vi "ProcessBufferUpdatesSubnet2.vi"(11 "MockFAILC2Settings":T1={"ModbusTxDataFIFO"="MockbusPort2TxFIFO", "Code17Memory"="MockFAILC2Code17", "BufferUpdateFIFO"="MockFAILC2Command", "ModbusRxDataFIFO"="MockbusPort2RxFIFO", "Code18Memory"="MockFAILC2Code18", "Code65Memory"="MockFAILC2Code65", "Code66Memory"="MockFAILC2Code66", "Code67Memory"="MockFAILC2Code67", "Code72Memory"="MockFAILC2Code72", "Code80Memory"="MockFAILC2Code80", "Code110Memory"="MockFAILC2Code110", "CRCDataFIFO"="MockFAILC2CRCDataFIFO", "CRCCalculateFIFO"="MockFAILC2CRCCalculateFIFO", "CRCFIFO"="MockFAILC2CRCFIFO"}) -> ()   [LabVIEW 2016]
uses:
  DataTypes/MockFAILC2Settings.ctl
  FPGAMockHPILC/DataTypes/MockHPBufferUpdateLoopData.ctl
  FPGAMockHPILC/DataTypes/MockHPBufferUpdateStates.ctl
  <vilib>/Platform/TimedLoop/XDataNode/timing_clust.ctl
  <vilib>/Platform/TimedLoop/XDataNode/nitl_modes.ctl
  <vilib>/Platform/TimedLoop/XDataNode/wakeup.ctl
  <vilib>/rvi/Emulation/niFpgaSctlEmulationGetInTimedLoop.vi
  <vilib>/rvi/Emulation/niFpgaEmulationReportErrorSimple.vi
  <vilib>/rvi/Emulation/niFpgaGetClockAttributes.vi
  <vilib>/rvi/Emulation/niFpgaCriticalErrorInLSC.vi
  <vilib>/rvi/DataTransferAndStorage/Container/Common/niFpgaContainerExecOnDevCompGetState.vi
  <vilib>/rvi/Emulation/niFpgaEmulationIsFPGAContextNoSignature.vi
  <vilib>/rvi/errors/niFpgaSetErrorForExecOnDevCompSimple.vi
  <vilib>/rvi/eio/common/nirviEmuReportErrorAndStop.vi
  <vilib>/rvi/DataTransferAndStorage/Container/Common/niFpgaContainerGetUniqueNameForEmu.vi
  <vilib>/rvi/FIFO/Fifo_Resource/nirvififoEmulationSetSize.vi
  <vilib>/rvi/FIFO/Fifo_Resource/nirviFifoEmulationQueueMgr.vi
  <instcachedir>/0/nirviFifoEmulationQueueMgr_E5CAEC123FF24DC58D834DCA3CDAA9B5.lvgen/nirviFifoEmulationQueueMgr_E5CAEC123FF24DC58D834DCA3CDAA9B5_009.vi
  <vilib>/rvi/FIFO/Fifo_Resource/nirvififoEmulationDetermineInputValidOut.vi
  <vilib>/rvi/FIFO/Fifo_Resource/nirvififoEmulationCreateLock.vi
  <vilib>/rvi/Emulation/niFpgaProcessEmulError.vi
  <vilib>/rvi/FIFO/Fifo_Resource/nirvififoEmulationObtainLock.vi
  <vilib>/rvi/FIFO/Fifo_Resource/nirvififoEmulationReleaseLock.vi
  <vilib>/rvi/occurrence/nirviWaitOnOccurrenceBase.vi
  <vilib>/rvi/errors/nirviReportUnexpectedCaseInternalError.vi
  <vilib>/rvi/errors/nirviReportUnexpectedCaseInternalError (U32).vi
  <vilib>/Utility/error.llb/Clear Errors.vi
  <vilib>/rvi/interface/RandomDataEmulation/niFpgaRandomDataHandleErrors.vi
  <vilib>/rvi/Memory/Memory_Emulation/niFpgaMemoryEmulationCacheClearOnFirstRun.vi
  <vilib>/rvi/Memory/Memory_Emulation/nirvimemoryEmulationManagerCache_MakeExclusive.vi
  <vilib>/rvi/Memory/Memory_Emulation/niFpgaMemoryEmulationValidateCache.vi
  <vilib>/rvi/Memory/Memory_Emulation/nirvimemoryEmulationManagerCache_InsertValue.vi
  <vilib>/rvi/Memory/Memory_Emulation/nirvimemoryEmulationManagerCache_ReleaseExclusive.vi
  <vilib>/rvi/Memory/Memory_Emulation/nirvimemoryEmulationManagerCache_GetValue.vi
  <vilib>/rvi/Memory/Memory_Emulation/nirvimemoryEmulationManagerCache_SetValue.vi
  <vilib>/rvi/Emulation/niFpgaSctlEmulationResourceMgr.vi
  <vilib>/Platform/TimedLoop/XDataNode/XDataNode.xnode
  <vilib>/rvi/DataTransferAndStorage/Container/XNode/niFpgaContainer.xnode
  <vilib>/rvi/FIFO/Fifo_Resource/niFpgaFifoEmulationRefIn.vi
  <vilib>/rvi/Memory/Memory_Emulation/niFpgaMemoryEmulationRefIn.vi
  <vilib>/Platform/TimedLoop/XDataNode/XDNodeRunTimeDep.lvlib
  FPGAMockHPILC/FPGAMockHPILC.lvlib
  FPGAMockFAILC.lvlib
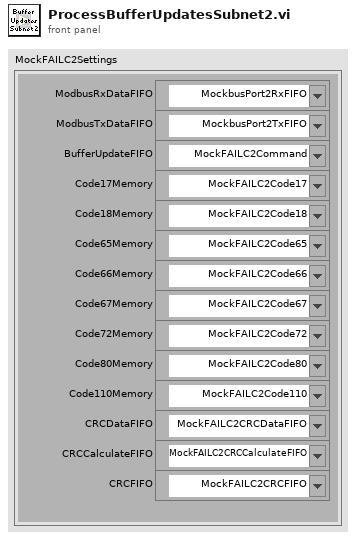
[diagram p1: front panel]
types:
  T1 = typedef "FPGAMockFAILC.lvlib/MockFAILC2Settings.ctl" = cluster{"ModbusTxDataFIFO":refnum<k21>, "Code17Memory":refnum<k21>, "BufferUpdateFIFO":refnum<k21>, "ModbusRxDataFIFO":refnum<k21>, "Code18Memory":refnum<k21>, "Code65Memory":refnum<k21>, "Code66Memory":refnum<k21>, "Code67Memory":refnum<k21>, "Code72Memory":refnum<k21>, "Code80Memory":refnum<k21>, "Code110Memory":refnum<k21>, "CRCDataFIFO":refnum<k21>, "CRCCalculateFIFO":refnum<k21>, "CRCFIFO":refnum<k21>}
  T2 = typedef "FPGAMockHPILC.lvlib/MockHPBufferUpdateLoopData.ctl" = cluster{"BufferUpdateLoopStates":T3, "Address":u8, "Function":u8, "Length":u8, "Data":u8, "Index":u8}
  T3 = typedef "FPGAMockHPILC.lvlib/MockHPBufferUpdateStates.ctl" = enum16{"ReadAddress", "ReadFunction", "ReadLength", "ReadData", "WriteData"}
  T4 = typedef "XDNodeRunTimeDep.lvlib/timing_clust.ctl" = cluster{"Expected End [f-1]":u64, "Actual End [f-1]":u64, "Finished Late? [f-1]":bool, "Expected End [i-1]":u64, "Actual End [i-1]":u64, "Finished Late? [i-1]":bool, "Expected Start [i]":u64, "Actual Start [i]":u64, "Expected Start [f]":u64, "Actual Start [f]":u64, "Source Name":string, "Structure Name":string, "Period":i64, "Deadline":i64, "Offset":i64, "Start":i64, "Priority":i32, "Timeout":i32, "Mode":T5, "Wakeup Reason":T6, "Error":errorcluster, "Source Type":string, "Secondary Source Type":string, "Global End Time":u64, "Global Start Time":u64, "Frame Duration":u64, "Iteration Duration":u64, "Assigned CPU":i32, "I/O Scan Engine Mode":u32}
  T5 = typedef "XDNodeRunTimeDep.lvlib/nitl_modes.ctl" = enum32{"No Change", "Process missed periods, maintain original phase", "Discard missed periods, maintain original phase", "Process missed periods, ignore original phase", "Discard missed periods, ignore original phase"}
  T6 = typedef "XDNodeRunTimeDep.lvlib/wakeup.ctl" = enum32{"Normal", "Aborted", "Asynchronous wakeup", "Timing source error", "Timed loop error", "Timeout"}
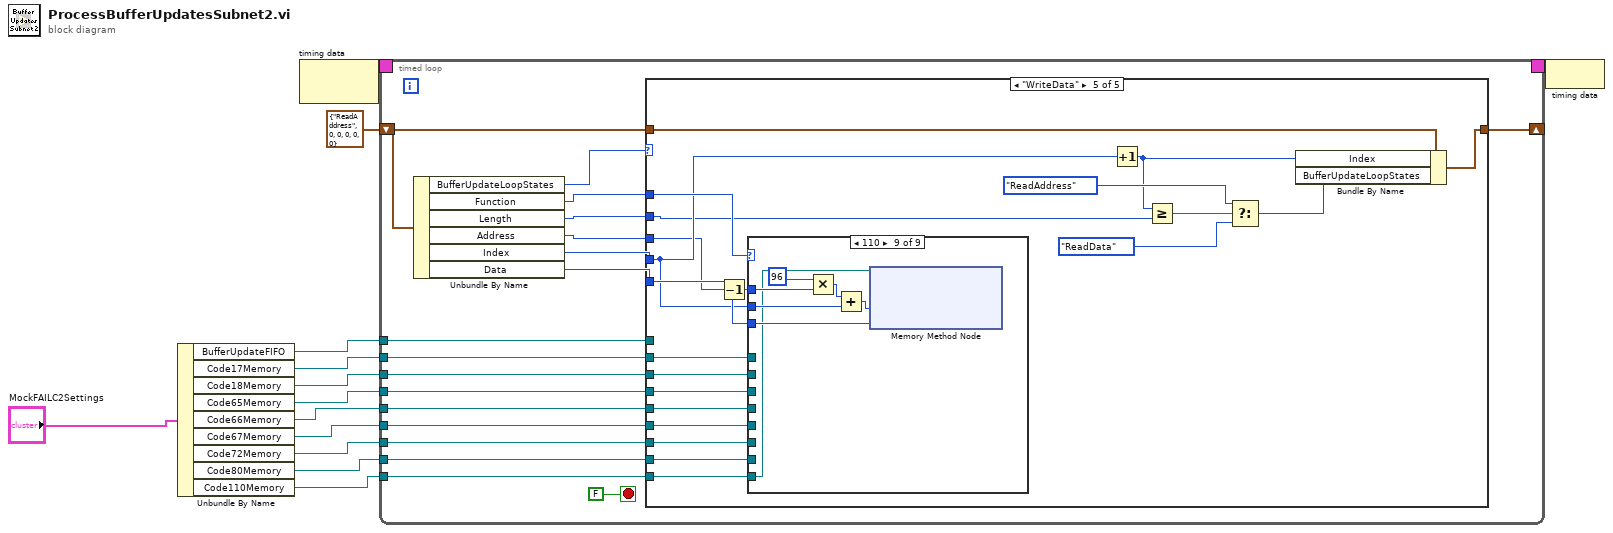
[diagram p0: block diagram]
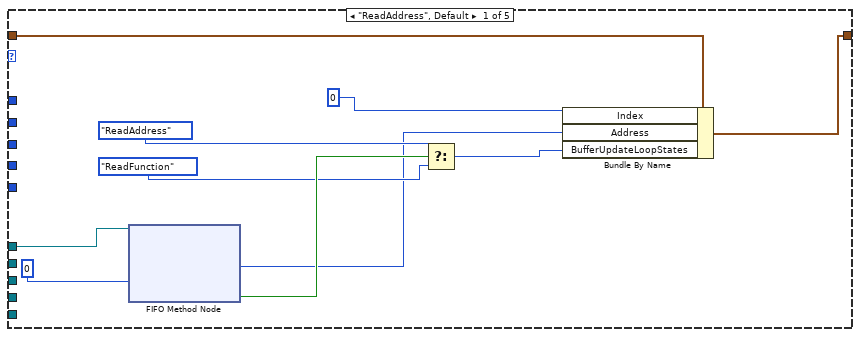
[diagram p2: hidden frame]
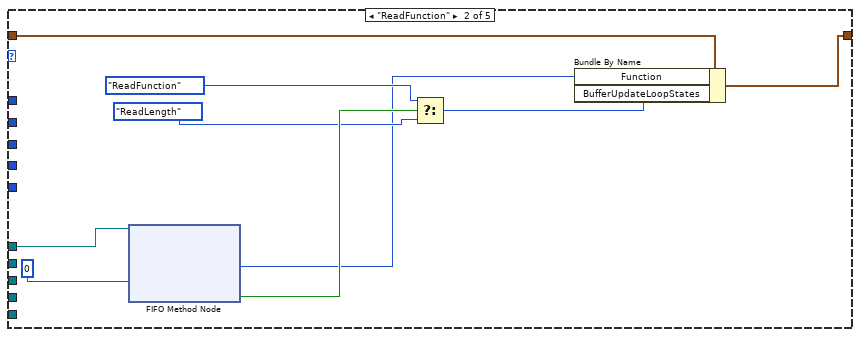
[diagram p3: hidden frame]
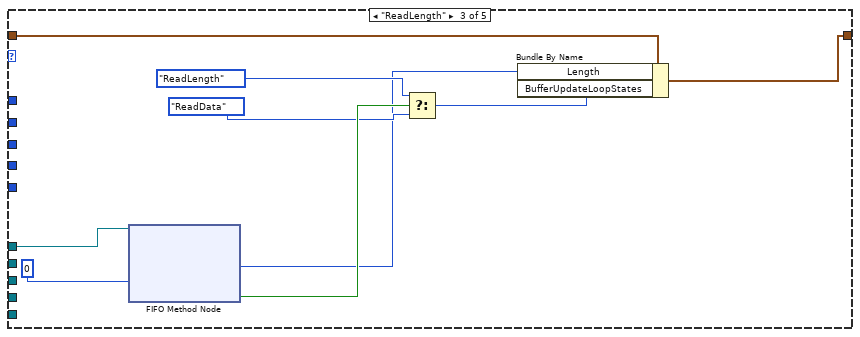
[diagram p4: hidden frame]
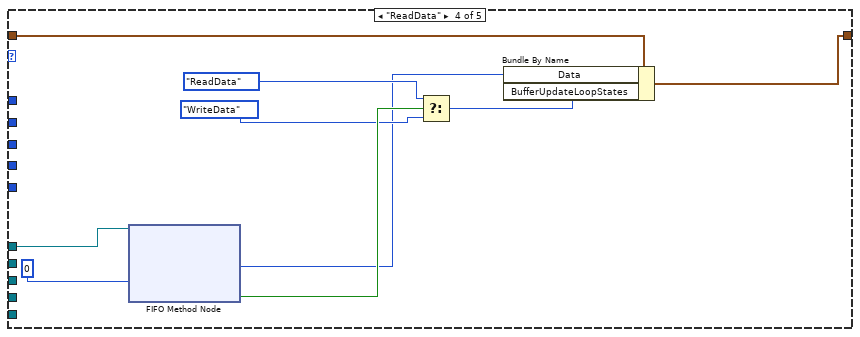
[diagram p5: hidden frame]
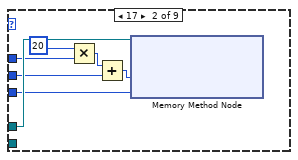
[diagram p7: hidden frame]
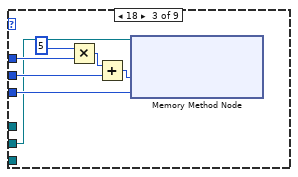
[diagram p8: hidden frame]
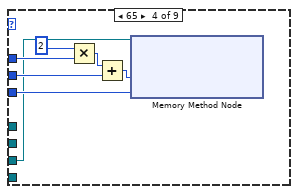
[diagram p9: hidden frame]
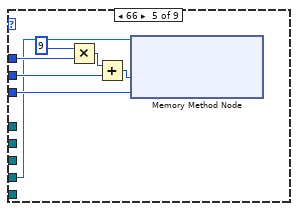
[diagram p10: hidden frame]
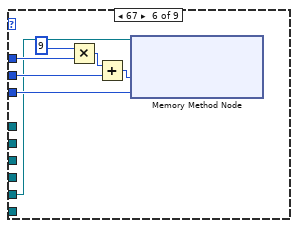
[diagram p11: hidden frame]
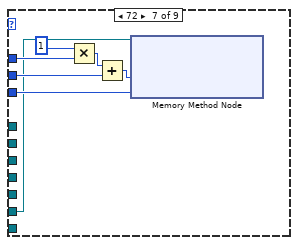
[diagram p12: hidden frame]
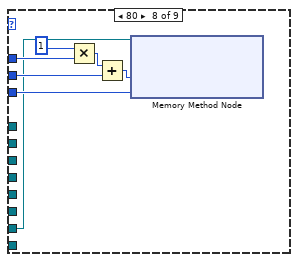
[diagram p13: hidden frame]
diagram:
  n1 = Unbundle By Name("MockFAILC2Settings") -> ("BufferUpdateFIFO"=w10:refnum<k21>, "Code17Memory"=w9:refnum<k21>, "Code18Memory"=w8:refnum<k21>, "Code65Memory"=w7:refnum<k21>, "Code66Memory"=w6:refnum<k21>, "Code67Memory"=w5:refnum<k21>, "Code72Memory"=w4:refnum<k21>, "Code80Memory"=w3:refnum<k21>, "Code110Memory"=w2:refnum<k21>)
  n2 = node-c288() -> (w13:T4)  [unwired: 1 in]
  n3 = timed-loop {
    timing: w13 -> [_]
    timing-out: [_] -> w12
    tunnel: w10 -> [w30]
    tunnel: w9 -> [w22]
    tunnel: w8 -> [w21]
    tunnel: w7 -> [w20]
    tunnel: w6 -> [w19]
    tunnel: w5 -> [w18]
    tunnel: w4 -> [w17]
    tunnel: w3 -> [w16]
    tunnel: w2 -> [w15]
    shift-right: [w24] -> _
    shift-left: T2 {"BufferUpdateLoopStates"=enum."ReadAddress", "Address"=0, "Function"=0, "Length"=0, "Data"=0, "Index"=0} ("MockHPBufferUpdateLoopData") -> [w29]
    stop <- FALSE stop-if-true
    n4 = Unbundle By Name(w29) -> ("BufferUpdateLoopStates"=w31:T3, "Function"=w28:u8, "Length"=w27:u8, "Address"=w26:u8, "Index"=w25:u8, "Data"=w23:u8)
    n5 = case shown="\"WriteData\"" w31 {
      tunnel: w30 -> [w41 w50 w59 w68 _]
      tunnel: w29 -> [w34 w43 w52 w61 w87]
      tunnel: w28 -> [_ _ _ _ w85]
      tunnel: w27 -> [_ _ _ _ w81]
      tunnel: w26 -> [_ _ _ _ w70]
      tunnel: w25 -> [_ _ _ _ w82]
      tunnel: [w33 w42 w51 w60 w86] -> w24
      tunnel: w23 -> [_ _ _ _ w83]
      tunnel: w22 -> [_ _ _ _ w84]
      tunnel: w21 -> [_ _ _ _ w77]
      tunnel: w20 -> [_ _ _ _ w76]
      tunnel: w19 -> [_ _ _ _ w75]
      tunnel: w18 -> [_ _ _ _ w74]
      tunnel: w17 -> [_ _ _ _ w73]
      tunnel: w16 -> [_ _ _ _ w72]
      tunnel: w15 -> [_ _ _ _ w71]
      frame "ReadAddress", Default {
        n6 = xnode ("FIFO Method Node")("Timeout"=0, "FIFO In"=w41) -> ("Element"=w36:u8, "Timed Out?"=w40:bool)  [unwired: 1 out]
        n7 = Select(t=MockHPBufferUpdateStates."ReadAddress" ("f"), s=w40, f=MockHPBufferUpdateStates."ReadFunction") -> (s? t:f=w35:T3)
        n8 = Bundle By Name(cluster=w34, "Index"=u8 0, "Address"=w36, "BufferUpdateLoopStates"=w35) -> (w33:T2)
      }
      frame "ReadFunction" {
        n9 = xnode ("FIFO Method Node")("Timeout"=0, "FIFO In"=w50) -> ("Element"=w45:u8, "Timed Out?"=w49:bool)  [unwired: 1 out]
        n10 = Select(t=MockHPBufferUpdateStates."ReadFunction" ("f"), s=w49, f=MockHPBufferUpdateStates."ReadLength") -> (s? t:f=w44:T3)
        n11 = Bundle By Name(cluster=w43, "Function"=w45, "BufferUpdateLoopStates"=w44) -> (w42:T2)
      }
      frame "ReadLength" {
        n12 = xnode ("FIFO Method Node")("Timeout"=0, "FIFO In"=w59) -> ("Element"=w54:u8, "Timed Out?"=w58:bool)  [unwired: 1 out]
        n13 = Select(t=MockHPBufferUpdateStates."ReadLength" ("f"), s=w58, f=MockHPBufferUpdateStates."ReadData") -> (s? t:f=w53:T3)
        n14 = Bundle By Name(cluster=w52, "Length"=w54, "BufferUpdateLoopStates"=w53) -> (w51:T2)
      }
      frame "ReadData" {
        n15 = xnode ("FIFO Method Node")("Timeout"=0, "FIFO In"=w68) -> ("Element"=w63:u8, "Timed Out?"=w67:bool)  [unwired: 1 out]
        n16 = Select(t=MockHPBufferUpdateStates."ReadData" ("f"), s=w67, f=MockHPBufferUpdateStates."WriteData") -> (s? t:f=w62:T3)
        n17 = Bundle By Name(cluster=w61, "Data"=w63, "BufferUpdateLoopStates"=w62) -> (w60:T2)
      }
      frame "WriteData" {
        n18 = Decrement(x=w70) -> (x-1=w69:u8)
        n19 = case shown="110" w85 {
          tunnel: w84 -> [_ w96 _ _ _ _ _ _ _]
          tunnel: w83 -> [_ w95 w103 w110 w117 w124 w131 w138 w145]
          tunnel: w82 -> [_ w93 w101 w108 w115 w122 w129 w136 w143]
          tunnel: w69 -> [_ w91 w99 w106 w113 w120 w127 w134 w141]
          tunnel: w77 -> [_ _ w97 _ _ _ _ _ _]
          tunnel: w76 -> [_ _ _ w104 _ _ _ _ _]
          tunnel: w75 -> [_ _ _ _ w111 _ _ _ _]
          tunnel: w74 -> [_ _ _ _ _ w118 _ _ _]
          tunnel: w73 -> [_ _ _ _ _ _ w125 _ _]
          tunnel: w72 -> [_ _ _ _ _ _ _ w132 _]
          tunnel: w71 -> [_ _ _ _ _ _ _ _ w139]
          frame 0, Default {
          }
          frame 17 {
            n20 = Multiply(x=u8 20, y=w91) -> (x*y=w94:u8)
            n21 = Add(x=w94, y=w93) -> (x+y=w92:u8)
            n22 = xnode ("Memory Method Node")("Address"=w92, "Data"=w95, "Memory In"=w96) -> ()  [unwired: 1 out]
          }
          frame 18 {
            n23 = Multiply(x=u8 5, y=w99) -> (x*y=w102:u8)
            n24 = Add(x=w102, y=w101) -> (x+y=w100:u8)
            n25 = xnode ("Memory Method Node")("Address"=w100, "Data"=w103, "Memory In"=w97) -> ()  [unwired: 1 out]
          }
          frame 65 {
            n26 = Multiply(x=u8 2, y=w106) -> (x*y=w109:u8)
            n27 = Add(x=w109, y=w108) -> (x+y=w107:u8)
            n28 = xnode ("Memory Method Node")("Address"=w107, "Data"=w110, "Memory In"=w104) -> ()  [unwired: 1 out]
          }
          frame 66 {
            n29 = Multiply(x=u8 9, y=w113) -> (x*y=w116:u8)
            n30 = Add(x=w116, y=w115) -> (x+y=w114:u8)
            n31 = xnode ("Memory Method Node")("Address"=w114, "Data"=w117, "Memory In"=w111) -> ()  [unwired: 1 out]
          }
          frame 67 {
            n32 = Multiply(x=u8 9, y=w120) -> (x*y=w123:u8)
            n33 = Add(x=w123, y=w122) -> (x+y=w121:u8)
            n34 = xnode ("Memory Method Node")("Address"=w121, "Data"=w124, "Memory In"=w118) -> ()  [unwired: 1 out]
          }
          frame 72 {
            n35 = Multiply(x=u8 1, y=w127) -> (x*y=w130:u8)
            n36 = Add(x=w130, y=w129) -> (x+y=w128:u8)
            n37 = xnode ("Memory Method Node")("Address"=w128, "Data"=w131, "Memory In"=w125) -> ()  [unwired: 1 out]
          }
          frame 80 {
            n38 = Multiply(x=u8 1, y=w134) -> (x*y=w137:u8)
            n39 = Add(x=w137, y=w136) -> (x+y=w135:u8)
            n40 = xnode ("Memory Method Node")("Address"=w135, "Data"=w138, "Memory In"=w132) -> ()  [unwired: 1 out]
          }
          frame 110 {
            n41 = Multiply(x=u8 96, y=w141) -> (x*y=w144:u8)
            n42 = Add(x=w144, y=w143) -> (x+y=w142:u8)
            n43 = xnode ("Memory Method Node")("Address"=w142, "Data"=w145, "Memory In"=w139) -> ()  [unwired: 1 out]
          }
        }
        n44 = Increment(x=w82) -> (x+1=w78:u8)
        n45 = Greater Or Equal?(x=w78, y=w81) -> (x >= y?=w80:bool)
        n46 = Select(t=MockHPBufferUpdateStates."ReadAddress" ("f"), s=w80, f=MockHPBufferUpdateStates."ReadData") -> (s? t:f=w79:T3)
        n47 = Bundle By Name(cluster=w87, "Index"=w78, "BufferUpdateLoopStates"=w79) -> (w86:T2)
      }
    }
  }
  n48 = node-c288(w12) -> ()
